vi "PI_Feedforward.vi"(5 "Motor Effort Axis":dbl[](array[numeric]) format="%_6g", 6 "dT":dbl, 7 "Position Axis":dbl[](array[numeric]) format="%_6g", 9 "Control Inputs":T2={"Kp"=0.01, "Ki"=0.0, "i upper"=0.0, "i lower"=0.0, "Output upper"=1.0, "Output lower"=-1.0}, 10 "Feed Back":dbl, 11 "Target":dbl) -> (1 "Term Indicators":T1, 2 "Output":dbl, 3 "Error":dbl)   [LabVIEW 2014]
uses:
  <vilib>/gmath/NI_Gmath.lvlib
panel:
  in  "Deadband_Size(%)":dbl=9.0 format="%#_13g"
  in  "Deadband_Center":dbl=-0.00784 format="%#_13g"
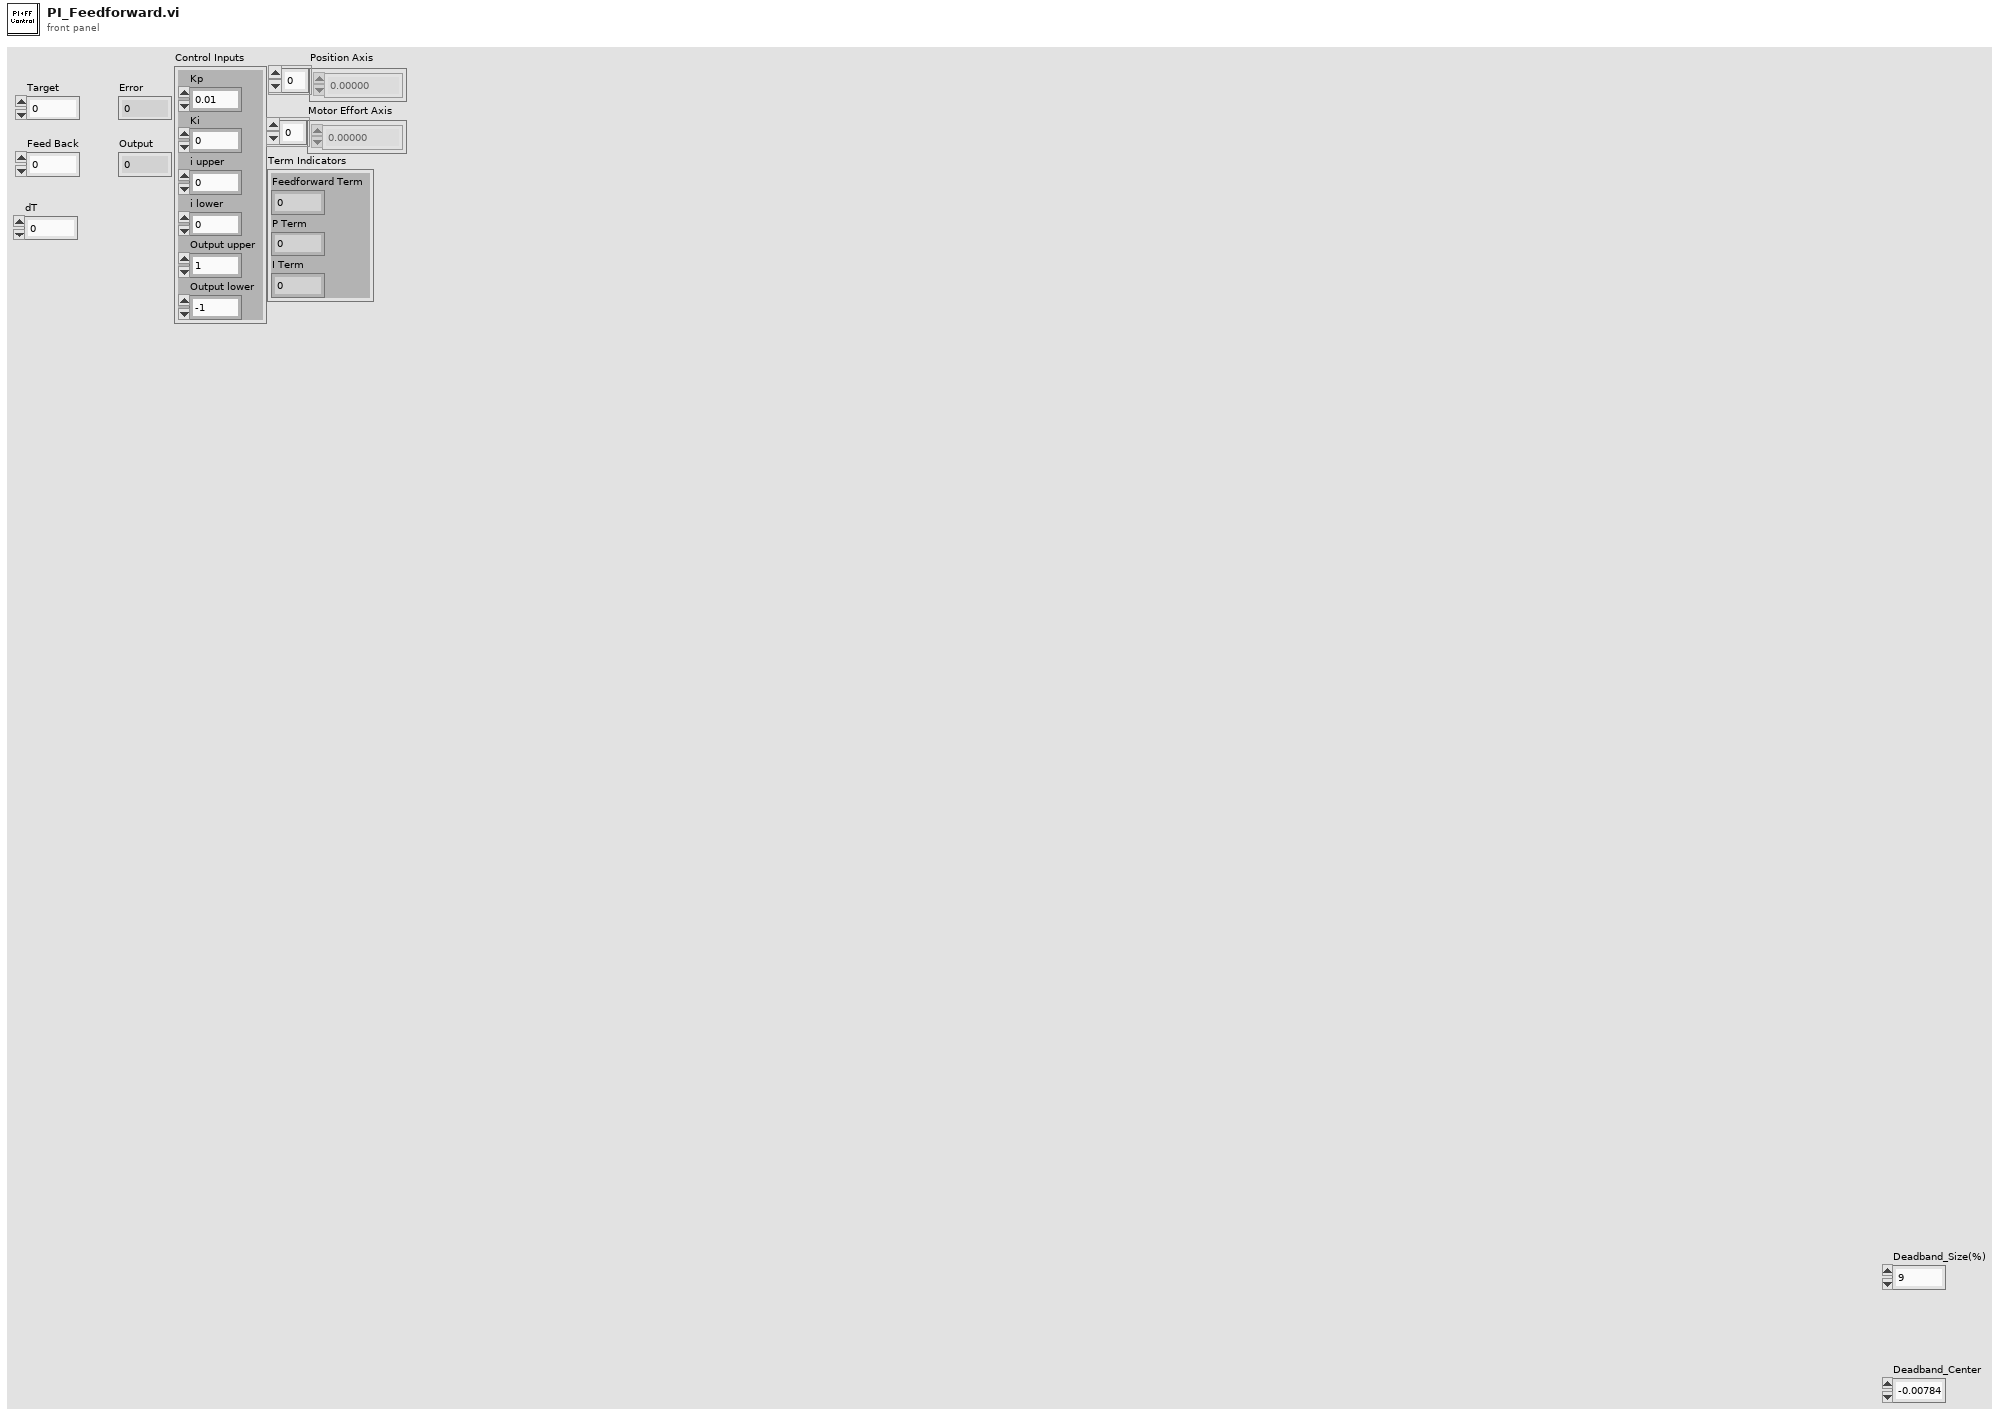
[diagram p1: front panel]
types:
  T1 = cluster{"Feedforward Term":dbl, "P Term ":dbl, "I Term":dbl}
  T2 = cluster{"Kp":dbl, "Ki":dbl, "i upper":dbl, "i lower":dbl, "Output upper":dbl, "Output lower":dbl}
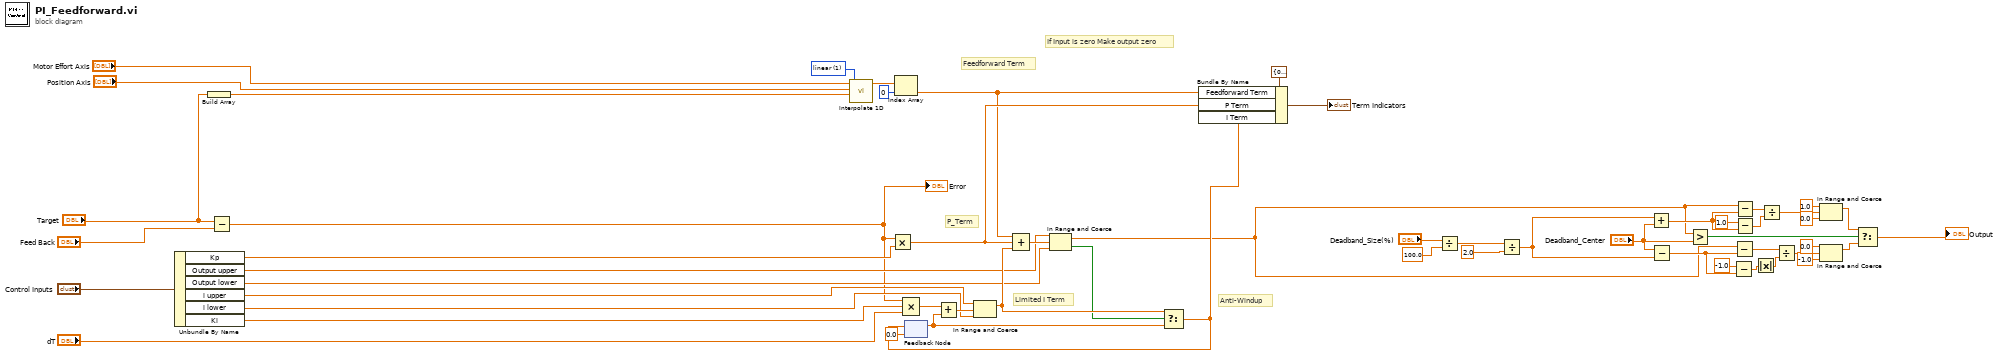
[diagram p0: block diagram]
diagram:
  w40 = 1 items=["nearest", "linear", "spline", "cubic Hermite", "Lagrange"] ("method")
  # "If Input is zero Make output zero"
  # "Feedforward Term"
  # "Anti-Windup"
  # "Limited I Term"
  # "P_Term"
  n1 = Unbundle By Name("Control Inputs") -> ("Kp"=w46:dbl, "Output upper"=w45:dbl, "Output lower"=w44:dbl, "i upper"=w43:dbl, "i lower"=w42:dbl, "Ki"=w41:dbl)
  n2 = Build Array("Target") -> (w39:dbl[])
  n3 = Subtract(x="Target", y="Feed Back") -> (x-y=w1:dbl)
  "Error" <- w1
  n4 = call <vilib>:"Interpolate 1D.vi"("method"=w40, "xi"=w39, "X"="Position Axis", "Y"="Motor Effort Axis") -> ("yi"=w36:dbl[])  [unwired: 5 in, 2 out]
  n5 = Multiply(x=w1, y=w46) -> (x*y=w32:dbl)
  n6 = Index Array(array=w36, index=0) -> (element=w30:dbl)
  n7 = Compound Arithmetic op=MULTIPLY(w1, w41, "dT") -> (w53:dbl)
  n8 = feedback #1(0.0 ("i upper")) -> (w49:dbl)
  n9 = Add(x=w53, y=w49) -> (x+y=w52:dbl)
  n10 = In Range and Coerce(upper limit=w43, x=w52, lower limit=w42) -> (coerced(x)=w50:dbl)  [unwired: 1 out]
  n11 = Compound Arithmetic op=ADD(w30, w32, w50) -> (w51:dbl)
  n12 = In Range and Coerce(upper limit=w45, x=w51, lower limit=w44) -> (coerced(x)=w2:dbl, In Range?=w48:bool)
  n13 = Select(t=w50, s=w48, f=w49) -> (s? t:f=w31:dbl)
  n14 = feedback-in #1(w31) -> ()
  n15 = Bundle By Name(cluster=T1 {"Feedforward Term"=0.0, "P Term "=0.0, "I Term"=0.0} ("Term Indicators"), "Feedforward Term"=w30, "P Term"=w32, "I Term"=w31) -> (→"Term Indicators":T1)
  n16 = Divide(x="Deadband_Size(%)", y=100.0) -> (x/y=w6:dbl)
  n17 = Divide(x=w6, y=2.0) -> (x/y=w7:dbl)
  n18 = Add(x=w7, y="Deadband_Center") -> (x+y=w10:dbl)
  n19 = Subtract(x="Deadband_Center", y=w7) -> (x-y=w19:dbl)
  n20 = Greater?(x=w2, y="Deadband_Center") -> (0:w25:bool)
  n21 = Subtract(x=-1.0, y=w19) -> (x-y=w26:dbl)
  n22 = Subtract(x=w2, y=w19) -> (x-y=w17:dbl)
  n23 = Subtract(x=w2, y=w10) -> (x-y=w11:dbl)
  n24 = Subtract(x=1.0, y=w10) -> (x-y=w12:dbl)
  n25 = Absolute Value(x=w26) -> (abs(x)=w27:dbl)
  n26 = Divide(x=w11, y=w12) -> (x/y=w15:dbl)
  n27 = Divide(x=w17, y=w27) -> (x/y=w20:dbl)
  n28 = In Range and Coerce(upper limit=1.0, x=w15, lower limit=0.0) -> (coerced(x)=w16:dbl)  [unwired: 1 out]
  n29 = In Range and Coerce(upper limit=0.0, x=w20, lower limit=-1.0) -> (coerced(x)=w23:dbl)  [unwired: 1 out]
  n30 = Select(t=w16, s=w25, f=w23) -> (s? t:f=→"Output":dbl)
